vi "Update-sender-activity.vi"(8 "error in (no error)":errorcluster, 10 "Message":refnum<class "Message.lvclass">, 11 "ModComm in":T1) -> (0 "error out":errorcluster, 2 "Message dup":refnum<class "Message.lvclass">, 3 "ModComm out":T1)   [LabVIEW 2013, in "SLMServer.lvlib" / "SLMServer.lvclass"]
uses:
  SLMServer.lvclass
  Object-reference.ctl
  SA-SLMAPI/Sources/Message.lvclass
  SA-SLMAPI/Sources/Message.lvclass/Message.ctl
  SA-SLMAPI/Sources/Read Sender ID.vi
  SA-SLMAPI/Sources/Read Send time.vi
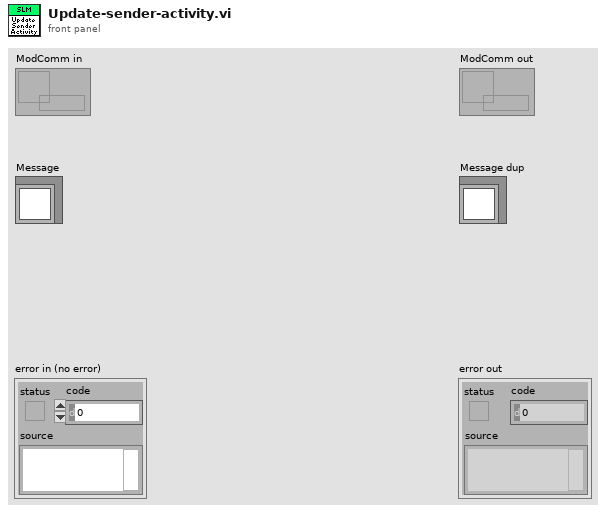
[diagram p1: front panel]
types:
  T1 = typedef "SLMServer.lvlib/SLMServer.lvclass/Object-reference.ctl" = refnum<data-value>
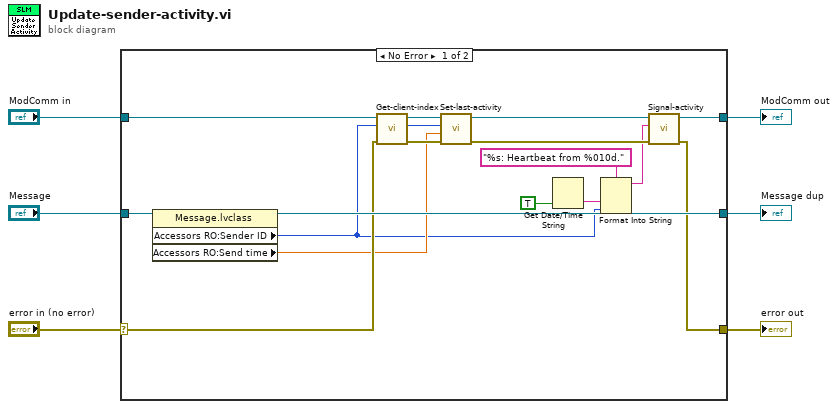
[diagram p0: block diagram]
diagram:
  n1 = case shown="No Error" "error in (no error)" {
    selector: "error in (no error)" -> [w19 w26]
    tunnel: [w12 w26] -> w5
    tunnel: [w14 w25] -> w3
    tunnel: "ModComm in" -> [w21 w25]
    tunnel: "Message" -> [w23 w24]
    tunnel: [w22 w24] -> w1
    frame No Error {
      n2 = property class="Message.lvclass"(reference=w23) -> (reference out=w22:refnum<class "Message.lvclass">, "Accessors RO:Sender ID"=w7:i32, "Accessors RO:Send time"=w16:dbl)  [unwired: 1 in, 1 out]
      n3 = call "Get-client-index.vi"("error in (no error)"=w19, "Client ID"=w7, "ModComm in"=w21) -> ("error out"=w18:errorcluster, "Client index"=w17:i32, "ModComm out"=w20:T1)  [unwired: 6 in]
      n4 = call "Set-last-activity.vi"("error in (no error)"=w18, "Last contact"=w16, "Client index"=w17, "ModComm in"=w20) -> ("error out"=w13:errorcluster, "ModComm out"=w15:T1)  [unwired: 6 in]
      n5 = Get Date/Time String(want seconds? (F)=TRUE) -> (time string=w8:string)  [unwired: 2 in, 1 out]
      n6 = Format Into String(format string="%s: Heartbeat from %010d.", w8, w7) -> (resulting string=w11:string)  [unwired: 2 in, 1 out]
      n7 = call "Signal-activity.vi"("error in (no error)"=w13, "Log message"=w11, "ModComm in"=w15) -> ("error out"=w12:errorcluster, "ModComm out"=w14:T1)  [unwired: 7 in]
    }
    frame Error {
    }
  }
  "error out" <- w5
  "ModComm out" <- w3
  "Message dup" <- w1
